vi "Import File - Tx Packet XML.vi"(6 "Root Node":refnum<k24>, 8 "error in (no error)":errorcluster) -> (0 "error out":errorcluster, 1 "Packet Header Data":T13, 4 "Tx Packet":T1 {"threadOptions"."pclDecimation" max=16 step=1; "threadOptions"."loopPeriod" max=16 step=1; "threadOptions"."targetPriority" min=-2 max=16 step=1; "threadOptions"."targetProcessor" min=-2 max=16 step=1; "Endianness" items=["big-endian"=0, "little-endian"=2]})   [LabVIEW 2019, in "UDP-Custom-Device System Explorer.lvlib"]
uses:
  UDP-Custom-Device System Explorer.lvlib
  System.Xml
  Types/XML - New/ImpExp - Packet Headers.ctl
  Types/XML - New/ImpExp - Tx Packet Data.ctl
  <vilib>/NI VeriStand/Custom Device API/Custom Device Item Info.ctl
  Shared/Types/Shared - Channel Data Type.ctl
  Shared/Types/Shared - Buffered.PacketInfo.ctl
  Shared/Types/Shared - Pointer Encoding.ctl
  Shared/Types/Shared - Receive Buffer Options.ctl
  Shared/Types/Shared - Transmit Buffer Options.ctl
  Shared/Types/Shared - Transmit Flag Options.ctl
  Shared/Types/Shared - Transmit Echo Options.ctl
  Types/Threading/Thread Configuration.ctl
  Types/Threading/Thread Sync Reference.ctl
  Shared/Types/Shared - Thread Management.ctl
  <vilib>/NI VeriStand/Custom Device API/Custom Device API.lvlib
  Shared/UDP-Custom-Device Shared.lvlib
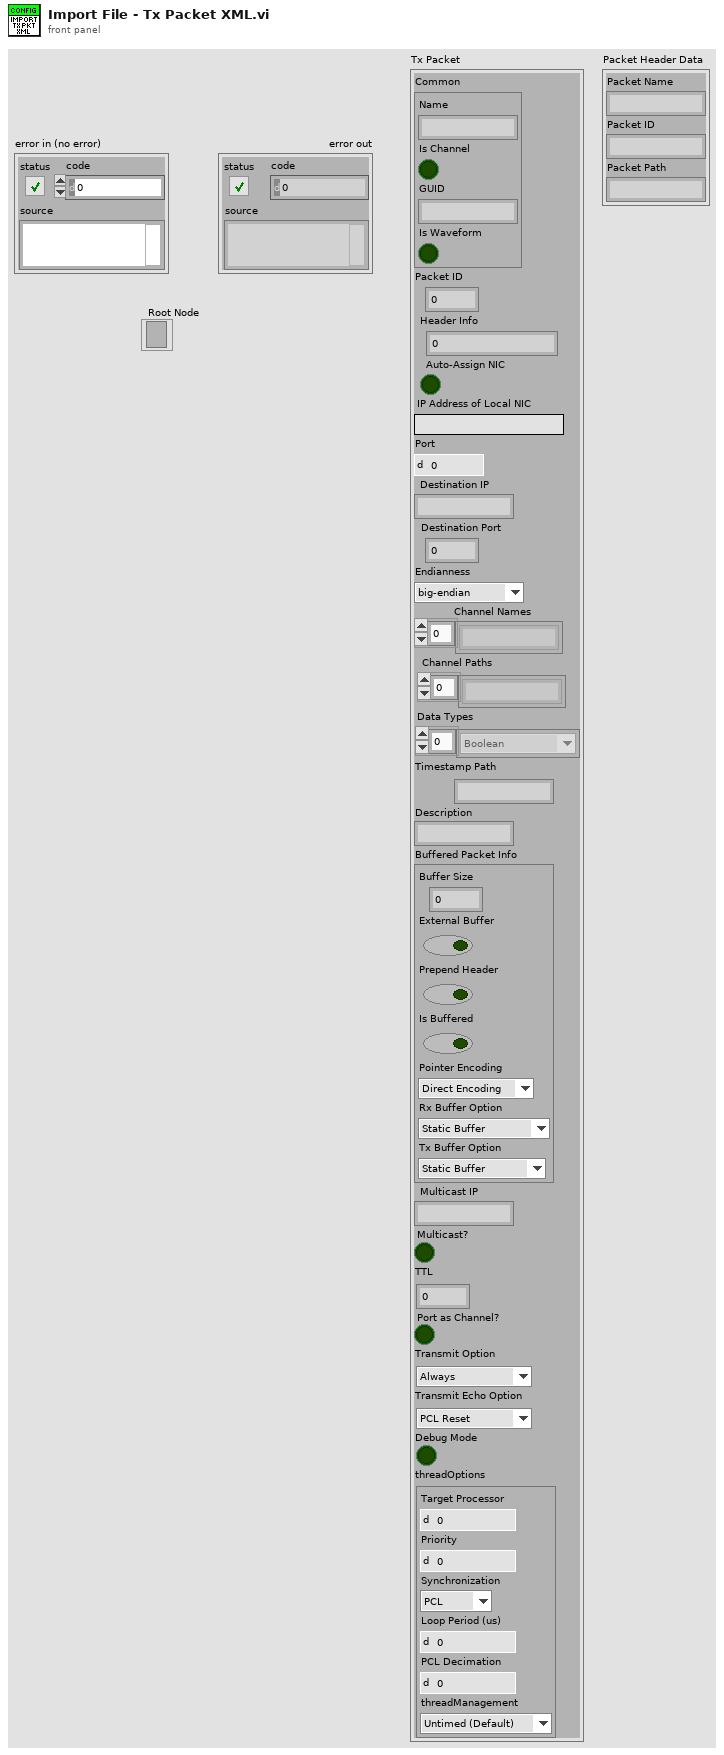
[diagram p1: front panel]
types:
  T1 = typedef "UDP-Custom-Device System Explorer.lvlib/ImpExp - Tx Packet Data.ctl" = cluster{"Common":T2, "Packet ID":i32, "Header Info":u32, "Auto-Assign NIC":bool, "IP Address of Local NIC":string, "Port":u16, "Destination IP":string, "Destination Port":u16, "Endianness":u16, "Channel Names":string[], "Channel Paths":string[], "Data Types":T3[], "Timestamp Path":string, "Description":string, "Buffered Packet Info":T4, "Multicast IP":string, "Multicast?":bool, "TTL":u16, "Port as Channel?":bool, "Transmit Option":T8, "Transmit Echo Option":T9, "Debug Mode":bool, "threadOptions":T10}
  T2 = typedef "Custom Device API.lvlib/Custom Device Item Info.ctl" = cluster{"Name":string, "Is Channel":bool, "GUID":string, "Is Waveform":bool}
  T3 = typedef "UDP-Custom-Device Shared.lvlib/Shared - Channel Data Type.ctl" = enum16{"Boolean", "Single", "Double", "I8", "I16", "I32", "I64", "U8", "U16", "U32", "U64"}
  T4 = typedef "UDP-Custom-Device Shared.lvlib/Shared - Buffered.PacketInfo.ctl" = cluster{"Buffer Size":i32, "External Buffer":bool, "Prepend Header":bool, "Is Buffered":bool, "Pointer Encoding":T5, "Rx Buffer Option":T6, "Tx Buffer Option":T7}
  T5 = typedef "UDP-Custom-Device Shared.lvlib/Shared - Pointer Encoding.ctl" = enum16{"Direct Encoding", "Conversion Encoding"}
  T6 = typedef "UDP-Custom-Device Shared.lvlib/Shared - Receive Buffer Options.ctl" = enum16{"Static Buffer", "Circular Buffer", "Circular Buffer + Size", "Internal Cache", "Internal Cache + Size", "Ping Pong", "Ping Pong + Size"}
  T7 = typedef "UDP-Custom-Device Shared.lvlib/Shared - Transmit Buffer Options.ctl" = enum16{"Static Buffer", "FIFO Buffer", "FIFO Buffer + Port"}
  T8 = typedef "UDP-Custom-Device Shared.lvlib/Shared - Transmit Flag Options.ctl" = enum16{"Always", "One-Shot", "Toggle"}
  T9 = typedef "UDP-Custom-Device Shared.lvlib/Shared - Transmit Echo Options.ctl" = enum16{"PCL Reset", "Counter", "Mirror"}
  T10 = typedef "UDP-Custom-Device System Explorer.lvlib/Thread Configuration.ctl" = cluster{"targetProcessor":i8, "targetPriority":i16, "Synchronization":T11, "loopPeriod":u32, "pclDecimation":u16, "threadManagement":T12}
  T11 = typedef "UDP-Custom-Device System Explorer.lvlib/Thread Sync Reference.ctl" = enum16{"PCL", "Async"}
  T12 = typedef "UDP-Custom-Device Shared.lvlib/Shared - Thread Management.ctl" = enum16{"Untimed (Default)", "Timed (High Priority)"}
  T13 = typedef "UDP-Custom-Device System Explorer.lvlib/ImpExp - Packet Headers.ctl" = cluster{"Packet Name":string, "Packet ID":string, "Packet Path":string}
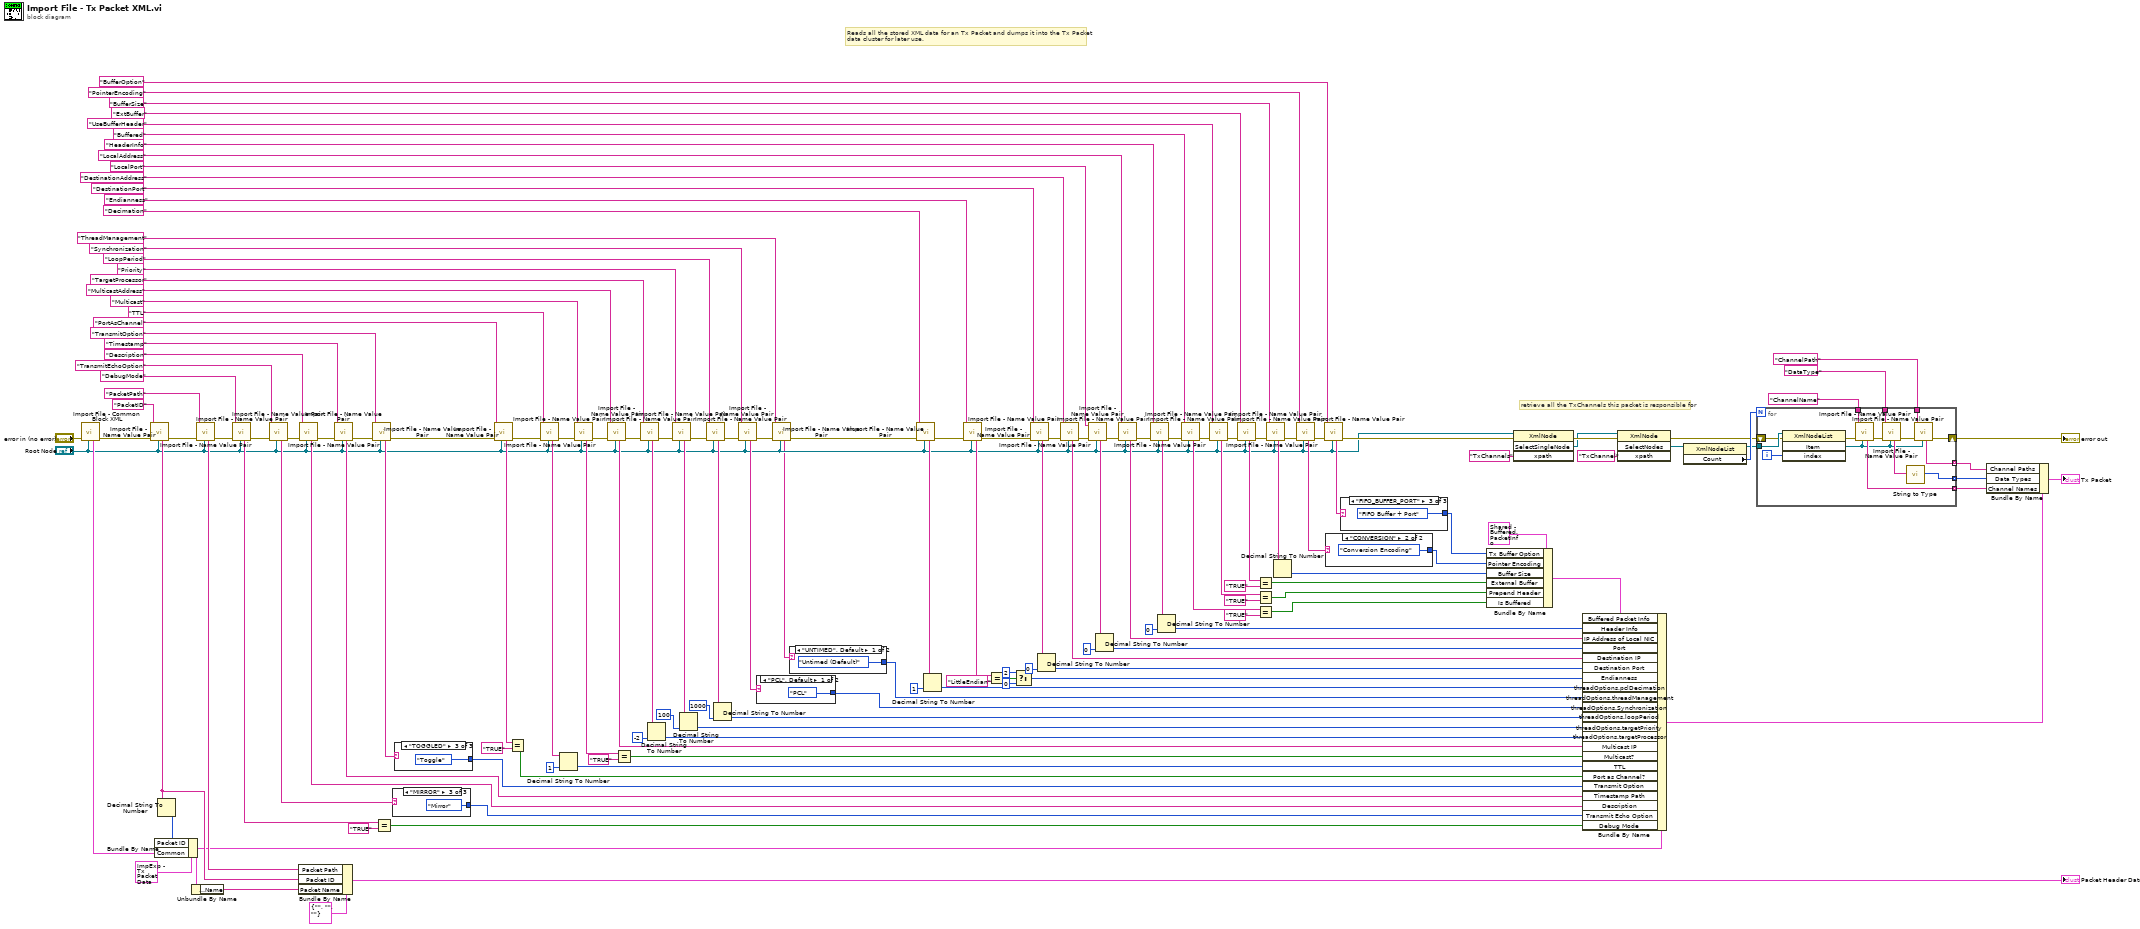
[diagram p0: block diagram]
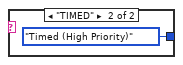
[diagram p2: hidden frame]
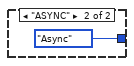
[diagram p3: hidden frame]
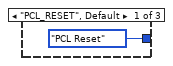
[diagram p4: hidden frame]
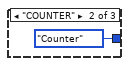
[diagram p5: hidden frame]
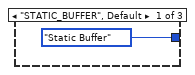
[diagram p6: hidden frame]
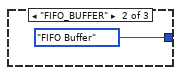
[diagram p7: hidden frame]
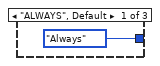
[diagram p8: hidden frame]
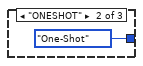
[diagram p9: hidden frame]
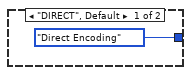
[diagram p10: hidden frame]
diagram:
  # "Reads all the stored XML data for an Tx Packet and dumps it into the Tx Packet\ndata cluster for later use."
  # "retrieve all the TxChannels this packet is responsible for"
  n1 = call "Import File - Common Block XML.vi"("Root Node"="Root Node", "error in (no error)"="error in (no error)") -> ("error out"=w150:errorcluster, "Common"=w154:T2)  [unwired: 8 in]
  n2 = call "Import File - Name Value Pair.vi"("Root Node"="Root Node", "error in (no error)"=w150, "Node Name"="PacketID") -> ("error out"=w147:errorcluster, "Value"=w145:string)  [unwired: 7 in]
  n3 = Decimal String To Number(string=w145) -> (number=w146:i32)  [unwired: 2 in, 1 out]
  n4 = Bundle By Name(cluster=T1 {"Common"={"Name"="", "Is Channel"=FALSE, "GUID"="", "Is Waveform"=FALSE}, "Packet ID"=0, "Header Info"=0, "Auto-Assign NIC"=FALSE, "IP Address of Local NIC"="", "Port"=0, "Destination IP"="", "Destination Port"=0, "Endianness"=0, "Channel Names"=[], "Channel Paths"=[], "Data Types"=[], "Timestamp Path"="", "Description"="", "Buffered Packet Info"={"Buffer Size"=0, "External Buffer"=FALSE, "Prepend Header"=FALSE, "Is Buffered"=FALSE, "Pointer Encoding"=enum."Direct Encoding", "Rx Buffer Option"=enum."Static Buffer", "Tx Buffer Option"=enum."Static Buffer"}, "Multicast IP"="", "Multicast?"=FALSE, "TTL"=0, "Port as Channel?"=FALSE, "Transmit Option"=enum."Always", "Transmit Echo Option"=enum."PCL Reset", "Debug Mode"=FALSE, "threadOptions"={"targetProcessor"=0, "targetPriority"=0, "Synchronization"=enum."PCL", "loopPeriod"=0, "pclDecimation"=0, "threadManagement"=enum."Untimed (Default)"}} ("Tx Packet"), "Packet ID"=w146, "Common"=w154) -> (w1:T1)
  n5 = Unbundle By Name(w1) -> ("Common.Name"=w152:string)
  n6 = call "Import File - Name Value Pair.vi"("Root Node"="Root Node", "error in (no error)"=w147, "Node Name"="PacketPath") -> ("error out"=w36:errorcluster, "Value"=w144:string)  [unwired: 7 in]
  n7 = call "Import File - Name Value Pair.vi"("Root Node"="Root Node", "error in (no error)"=w36, "Node Name"="DebugMode" ("Tag Name")) -> ("error out"=w35:errorcluster, "Value"=w32:string)  [unwired: 7 in]
  n8 = call "Import File - Name Value Pair.vi"("Root Node"="Root Node", "error in (no error)"=w35, "Node Name"="TransmitEchoOption" ("Tag Name")) -> ("error out"=w40:errorcluster, "Value"=w38:string)  [unwired: 7 in]
  n9 = Bundle By Name(cluster=T13 {"Packet Name"="", "Packet ID"="", "Packet Path"=""} ("Packet Header Data"), "Packet Path"=w144, "Packet ID"=w145, "Packet Name"=w152) -> (→"Packet Header Data":T13)
  n10 = call "Import File - Name Value Pair.vi"("Root Node"="Root Node", "error in (no error)"=w40, "Node Name"="Description") -> ("error out"=w142:errorcluster, "Value"=w13:string)  [unwired: 7 in]
  n11 = call "Import File - Name Value Pair.vi"("Root Node"="Root Node", "error in (no error)"=w142, "Node Name"="Timestamp") -> ("error out"=w48:errorcluster, "Value"=w14:string)  [unwired: 7 in]
  n12 = call "Import File - Name Value Pair.vi"("Root Node"="Root Node", "error in (no error)"=w48, "Node Name"="TransmitOption" ("Tag Name")) -> ("error out"=w47:errorcluster, "Value"=w46:string)  [unwired: 7 in]
  n13 = Equal?(x=w32, y="TRUE") -> (x = y?=w31:bool)
  n14 = case shown="\"MIRROR\"" w38 {
    tunnel: [Shared_-_Transmit_Echo_Options."PCL Reset" ("Transmit Echo Option") Shared_-_Transmit_Echo_Options."Counter" ("Transmit Echo Option") Shared_-_Transmit_Echo_Options."Mirror" ("Transmit Echo Option")] -> w37
    frame "PCL_RESET", Default {
    }
    frame "COUNTER" {
    }
    frame "MIRROR" {
    }
  }
  n15 = case shown="\"TOGGLED\"" w46 {
    tunnel: [Shared_-_Transmit_Flag_Options."Always" ("Transmit Options") Shared_-_Transmit_Flag_Options."One-Shot" ("Transmit Options") Shared_-_Transmit_Flag_Options."Toggle" ("Transmit Options")] -> w45
    frame "ALWAYS", Default {
    }
    frame "ONESHOT" {
    }
    frame "TOGGLED" {
    }
  }
  n16 = call "Import File - Name Value Pair.vi"("Root Node"="Root Node", "error in (no error)"=w47, "Node Name"="PortAsChannel" ("Tag Name")) -> ("error out"=w54:errorcluster, "Value"=w51:string)  [unwired: 7 in]
  n17 = Equal?(x=w51, y="TRUE") -> (x = y?=w50:bool)
  n18 = call "Import File - Name Value Pair.vi"("Root Node"="Root Node", "error in (no error)"=w54, "Node Name"="TTL" ("Tag Name")) -> ("error out"=w69:errorcluster, "Value"=w60:string)  [unwired: 7 in]
  n19 = Decimal String To Number(string=w60, default (0L)=u16 1 ("default (0 I32)")) -> (number=w59:u16)  [unwired: 1 in, 1 out]
  n20 = call "Import File - Name Value Pair.vi"("Root Node"="Root Node", "error in (no error)"=w69, "Node Name"="Multicast" ("Tag Name")) -> ("error out"=w70:errorcluster, "Value"=w63:string)  [unwired: 7 in]
  n21 = call "Import File - Name Value Pair.vi"("Root Node"="Root Node", "error in (no error)"=w70, "Node Name"="MulticastAddress" ("Tag Name")) -> ("error out"=w25:errorcluster, "Value"=w65:string)  [unwired: 7 in]
  n22 = Equal?(x=w63, y="TRUE") -> (x = y?=w62:bool)
  n23 = call "Import File - Name Value Pair.vi"("Root Node"="Root Node", "error in (no error)"=w25, "Node Name"="TargetProcessor" ("Tag Name")) -> ("error out"=w28:errorcluster, "Value"=w20:string)  [unwired: 7 in]
  n24 = Decimal String To Number(string=w20, default (0L)=i8 -2 ("default (0 I32)")) -> (number=w17:i8)  [unwired: 1 in, 1 out]
  n25 = call "Import File - Name Value Pair.vi"("Root Node"="Root Node", "error in (no error)"=w28, "Node Name"="Priority" ("Tag Name")) -> ("error out"=w27:errorcluster, "Value"=w19:string)  [unwired: 7 in]
  n26 = Decimal String To Number(string=w19, default (0L)=i16 100 ("default (0 I32)")) -> (number=w16:i16)  [unwired: 1 in, 1 out]
  n27 = call "Import File - Name Value Pair.vi"("Root Node"="Root Node", "error in (no error)"=w27, "Node Name"="LoopPeriod" ("Tag Name")) -> ("error out"=w26:errorcluster, "Value"=w18:string)  [unwired: 7 in]
  n28 = Decimal String To Number(string=w18, default (0L)=u32 1000 ("default (0 I32)")) -> (number=w15:u32)  [unwired: 1 in, 1 out]
  n29 = call "Import File - Name Value Pair.vi"("Root Node"="Root Node", "error in (no error)"=w26, "Node Name"="Synchronization" ("Tag Name")) -> ("error out"=w7:errorcluster, "Value"=w9:string)  [unwired: 7 in]
  n30 = case shown="\"PCL\", Default" w9 {
    tunnel: [Thread_Sync_Reference."PCL" ("threadOptions.Synchronization") Thread_Sync_Reference."Async" ("threadOptions.Synchronization")] -> w8
    frame "PCL", Default {
    }
    frame "ASYNC" {
    }
  }
  n31 = call "Import File - Name Value Pair.vi"("Root Node"="Root Node", "error in (no error)"=w7, "Node Name"="ThreadManagement" ("Tag Name")) -> ("error out"=w6:errorcluster, "Value"=w3:string)  [unwired: 7 in]
  n32 = case shown="\"UNTIMED\", Default" w3 {
    tunnel: [Shared_-_Thread_Management."Untimed (Default)" ("Thread Management") Shared_-_Thread_Management."Timed (High Priority)" ("Thread Management")] -> w2
    frame "UNTIMED", Default {
    }
    frame "TIMED" {
    }
  }
  n33 = call "Import File - Name Value Pair.vi"("Root Node"="Root Node", "error in (no error)"=w6, "Node Name"="Decimation") -> ("error out"=w117:errorcluster, "Value"=w118:string)  [unwired: 7 in]
  n34 = Decimal String To Number(string=w118, default (0L)=u16 1 ("Decimation")) -> (number=w29:u16)  [unwired: 1 in, 1 out]
  n35 = call "Import File - Name Value Pair.vi"("Root Node"="Root Node", "error in (no error)"=w117, "Node Name"="Endianness") -> ("error out"=w116:errorcluster, "Value"=w112:string)  [unwired: 7 in]
  n36 = Equal?(x=w112, y="LittleEndian") -> (x = y?=w114:bool)
  n37 = Select(t=u16 2 ("Endianness"), s=w114, f=u16 0 ("Endianness")) -> (s? t:f=w110:u16)
  n38 = call "Import File - Name Value Pair.vi"("Root Node"="Root Node", "error in (no error)"=w116, "Node Name"="DestinationPort") -> ("error out"=w138:errorcluster, "Value"=w108:string)  [unwired: 7 in]
  n39 = Decimal String To Number(string=w108, default (0L)=u16 0 ("default (0 I32)")) -> (number=w107:u16)  [unwired: 1 in, 1 out]
  n40 = call "Import File - Name Value Pair.vi"("Root Node"="Root Node", "error in (no error)"=w138, "Node Name"="DestinationAddress") -> ("error out"=w135:errorcluster, "Value"=w105:string)  [unwired: 7 in]
  n41 = call "Import File - Name Value Pair.vi"("Root Node"="Root Node", "error in (no error)"=w135, "Node Name"="LocalPort") -> ("error out"=w134:errorcluster, "Value"=w103:string)  [unwired: 7 in]
  n42 = Decimal String To Number(string=w103, default (0L)=u16 0 ("default (0 I32)")) -> (number=w102:u16)  [unwired: 1 in, 1 out]
  n43 = call "Import File - Name Value Pair.vi"("Root Node"="Root Node", "error in (no error)"=w134, "Node Name"="LocalAddress") -> ("error out"=w133:errorcluster, "Value"=w101:string)  [unwired: 7 in]
  n44 = call "Import File - Name Value Pair.vi"("Root Node"="Root Node", "error in (no error)"=w133, "Node Name"="HeaderInfo") -> ("error out"=w132:errorcluster, "Value"=w99:string)  [unwired: 7 in]
  n45 = Decimal String To Number(string=w99, default (0L)=u32 0 ("default (0 I32)")) -> (number=w98:u32)  [unwired: 1 in, 1 out]
  n46 = call "Import File - Name Value Pair.vi"("Root Node"="Root Node", "error in (no error)"=w132, "Node Name"="Buffered") -> ("error out"=w125:errorcluster, "Value"=w96:string)  [unwired: 7 in]
  n47 = call "Import File - Name Value Pair.vi"("Root Node"="Root Node", "error in (no error)"=w125, "Node Name"="UseBufferHeader") -> ("error out"=w124:errorcluster, "Value"=w93:string)  [unwired: 7 in]
  n48 = call "Import File - Name Value Pair.vi"("Root Node"="Root Node", "error in (no error)"=w124, "Node Name"="ExtBuffer") -> ("error out"=w123:errorcluster, "Value"=w92:string)  [unwired: 7 in]
  n49 = Equal?(x=w92, y="TRUE") -> (x = y?=w88:bool)
  n50 = Equal?(x=w93, y="TRUE") -> (x = y?=w89:bool)
  n51 = Equal?(x=w96, y="TRUE") -> (x = y?=w90:bool)
  n52 = call "Import File - Name Value Pair.vi"("Root Node"="Root Node", "error in (no error)"=w123, "Node Name"="BufferSize") -> ("error out"=w58:errorcluster, "Value"=w91:string)  [unwired: 7 in]
  n53 = Decimal String To Number(string=w91) -> (number=w87:i32)  [unwired: 2 in, 1 out]
  n54 = call "Import File - Name Value Pair.vi"("Root Node"="Root Node", "error in (no error)"=w58, "Node Name"="PointerEncoding" ("Tag Name")) -> ("error out"=w44:errorcluster, "Value"=w55:string)  [unwired: 7 in]
  n55 = call "Import File - Name Value Pair.vi"("Root Node"="Root Node", "error in (no error)"=w44, "Node Name"="BufferOption" ("Tag Name")) -> ("error out"=w43:errorcluster, "Value"=w42:string)  [unwired: 7 in]
  n56 = case shown="\"CONVERSION\"" w55 {
    tunnel: [Shared_-_Pointer_Encoding."Direct Encoding" ("Pointer Encoding") Shared_-_Pointer_Encoding."Conversion Encoding" ("Pointer Encoding")] -> w56
    frame "DIRECT", Default {
    }
    frame "CONVERSION" {
    }
  }
  n57 = case shown="\"FIFO_BUFFER_PORT\"" w42 {
    tunnel: [Shared_-_Transmit_Buffer_Options."Static Buffer" ("Buffer Option") Shared_-_Transmit_Buffer_Options."FIFO Buffer" ("Buffer Option") Shared_-_Transmit_Buffer_Options."FIFO Buffer + Port" ("Buffer Option")] -> w30
    frame "STATIC_BUFFER", Default {
    }
    frame "FIFO_BUFFER" {
    }
    frame "FIFO_BUFFER_PORT" {
    }
  }
  n58 = Bundle By Name(cluster=T4 {"Buffer Size"=0, "External Buffer"=FALSE, "Prepend Header"=FALSE, "Is Buffered"=FALSE, "Pointer Encoding"=enum."Direct Encoding", "Rx Buffer Option"=enum."Static Buffer", "Tx Buffer Option"=enum."Static Buffer"} ("Buffered Packet Info"), "Tx Buffer Option"=w30, "Pointer Encoding"=w56, "Buffer Size"=w87, "External Buffer"=w88, "Prepend Header"=w89, "Is Buffered"=w90) -> (w127:T4)
  n59 = invoke class="XmlNode" method="SelectSingleNode"(reference="Root Node", error in=w43, "xpath"="TxChannels") -> (error out=w86:errorcluster, "SelectSingleNode"=w85:refnum<k24>)  [unwired: 1 in, 2 out]
  n60 = Bundle By Name(cluster=w1, "Buffered Packet Info"=w127, "Header Info"=w98, "IP Address of Local NIC"=w101, "Port"=w102, "Destination IP"=w105, "Destination Port"=w107, "Endianness"=w110, "threadOptions.pclDecimation"=w29, "threadOptions.threadManagement"=w2, "threadOptions.Synchronization"=w8, "threadOptions.loopPeriod"=w15, "threadOptions.targetPriority"=w16, "threadOptions.targetProcessor"=w17, "Multicast IP"=w65, "Multicast?"=w62, "TTL"=w59, "Port as Channel?"=w50, "Transmit Option"=w45, "Timestamp Path"=w14, "Description"=w13, "Transmit Echo Option"=w37, "Debug Mode"=w31) -> (w126:T1)
  n61 = invoke class="XmlNode" method="SelectNodes"(reference=w85, error in=w86, "xpath"="TxChannel") -> (error out=w78:errorcluster, "SelectNodes"=w83:refnum<k24>)  [unwired: 1 in, 2 out]
  n62 = property class="XmlNodeList"(reference=w83) -> (reference out=w77:refnum<k24>, "Count"=w79:i32)  [unwired: 1 in, 1 out]
  n63 = for {
    N: w79 -> [_]
    shift-right: [w175] -> w71
    shift-left: w78 -> [w185]
    tunnel: w77 -> [w186]
    tunnel: "ChannelName" ("xpath") -> [w181]
    tunnel: "DataType" ("xpath") -> [w180]
    tunnel: [w179] -> w73 mode=indexing
    tunnel: [w177] -> w74 mode=indexing
    tunnel: "ChannelPath" ("xpath") -> [w174]
    tunnel: [w172] -> w75 mode=indexing
    i -> [w184]
    n64 = invoke class="XmlNodeList" method="Item"(reference=w186, error in=w185, "index"=w184) -> (error out=w183:errorcluster, "Item"=w173:refnum<k24>)  [unwired: 1 in, 2 out]
    n65 = call "Import File - Name Value Pair.vi"("Root Node"=w173, "error in (no error)"=w183, "Node Name"=w181) -> ("error out"=w182:errorcluster, "Value"=w179:string)  [unwired: 7 in]
    n66 = call "Import File - Name Value Pair.vi"("Root Node"=w173, "error in (no error)"=w182, "Node Name"=w180) -> ("error out"=w176:errorcluster, "Value"=w178:string)  [unwired: 7 in]
    n67 = call "String to Type.vi"("String Type"=w178) -> ("Data Type"=w177:T3)  [unwired: 10 in]
    n68 = call "Import File - Name Value Pair.vi"("Root Node"=w173, "error in (no error)"=w176, "Node Name"=w174) -> ("error out"=w175:errorcluster, "Value"=w172:string)  [unwired: 7 in]
  }
  "error out" <- w71
  n69 = Bundle By Name(cluster=w126, "Channel Paths"=w75, "Data Types"=w74, "Channel Names"=w73) -> (→"Tx Packet":T1)
